vi "tsfifo_clear_lin_receive_buffers.vi"(8 "error in (no error)":errorcluster caption="错误输入（无错误）", 10 "AIdxChn":i32, 11 "路径输入":path) -> (0 "error out":errorcluster caption="错误输出", 2 "return":i32, 3 "路径输出":path)   [LabVIEW 2014]
doc: "Function Introduction :\nClear the receiving buffer cache of LIN module\nCall location :\nCall this function to clear the LIN cache\nData, ensure that the received data is up-to-date\ninput parameter :\nAChn: LIN channel number that needs to clear cache\nReturn value :\n==0: Clear successfully\nOther values: Clearing failed"
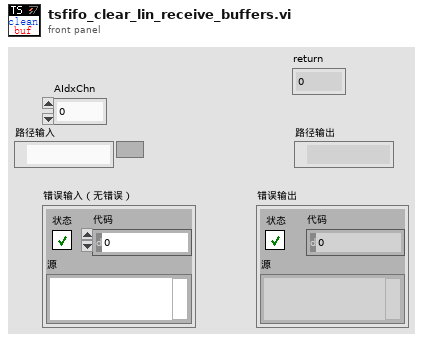
[diagram p1: front panel]
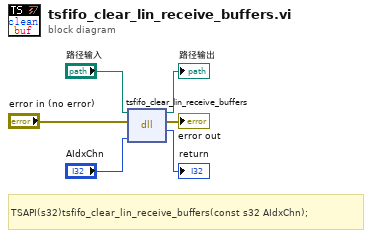
[diagram p0: block diagram]
diagram:
  # "TSAPI(s32)tsfifo_clear_lin_receive_buffers(const s32 AIdxChn);"
  n1 = dll-call lib="D:/Program Files (x86)/TOSUN/TSMaster/Data/SDK/lib/x86/TSMaster.*" fn="tsfifo_clear_lin_receive_buffers"(path in="路径输入", error in="error in (no error)", "AIdxChn"="AIdxChn") -> (path out=→"路径输出":path, error out=→"error out":errorcluster, "返回类型"=→"return":i32)  [unwired: 2 in]
